vi "SaveImagesFromArray (SubVI).vi"(8 "error in (no error)":errorcluster, 9 "Array of Images":T1[](array[typedef]), 10 "XY Camera Coordinates":dbl[][](array[numeric]), 11 "Path to save collected images":path=path "E:/XYZstage+Camera_CollectedImages/12-17-2016/images") -> (0 "error out":errorcluster)   [LabVIEW 2016]
uses:
  <vilib>/vision/Image Controls.llb/IMAQ Image.ctl
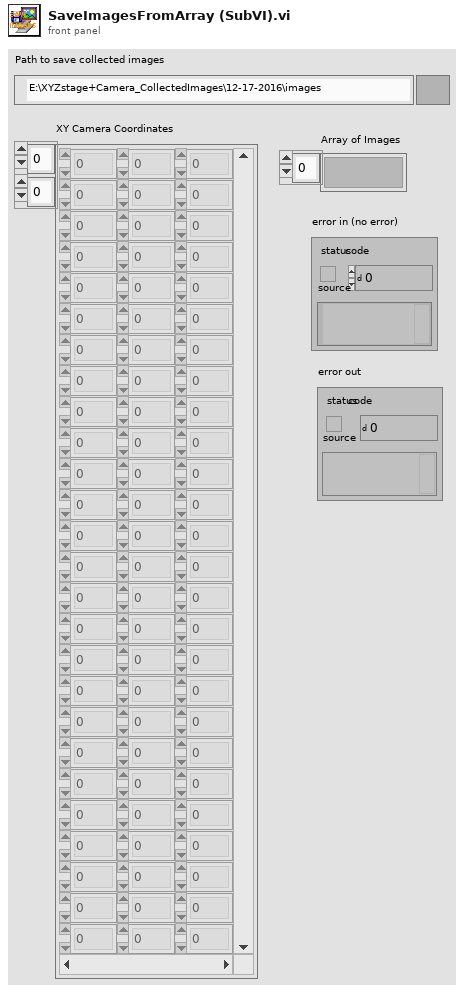
[diagram p1: front panel]
types:
  T1 = typedef "IMAQ Image.ctl" = refnum<image>
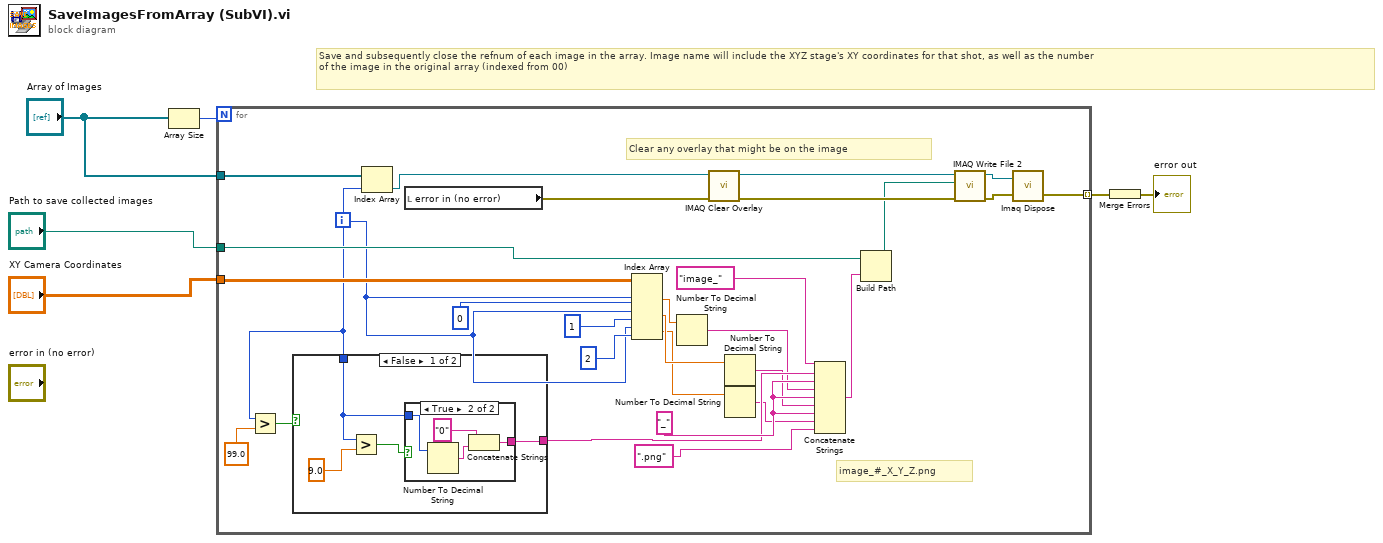
[diagram p0: block diagram]
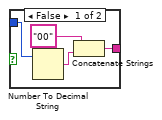
[diagram p2: hidden frame]
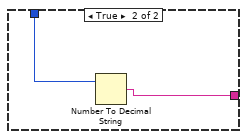
[diagram p3: hidden frame]
diagram:
  # "Save and subsequently close the refnum of each image in the array. Image name will include the XYZ stage's XY coordinates for that shot, as well as the number\nof the image in the original array (indexed from 00)"
  n1 = Array Size(array="Array of Images") -> (size(s)=w3:i32)
  n2 = for {
    N: w3 -> [_]
    tunnel: "Array of Images" -> [w34]
    tunnel: "Path to save collected images" -> [w27]
    tunnel: "XY Camera Coordinates" -> [w26]
    tunnel: [w23] -> w2 mode=indexing
    i -> [w7]
    w14 = "_" ("string")
    # "image_#_X_Y_Z.png"
    # "Clear any overlay that might be on the image"
    n3 = Greater?(x=w7, y=99.0) -> (0:w9:bool)
    n4 = case shown="False" w9 {
      tunnel: w7 -> [w35 w48]
      tunnel: [w37 w47] -> w13
      frame False {
        n5 = Greater?(x=w35, y=9.0) -> (0:w36:bool)
        n6 = case shown="True" w36 {
          tunnel: [w40 w43] -> w37
          tunnel: w35 -> [w39 w44]
          frame False {
            n7 = Number To Decimal String(number=w39) -> (decimal integer string=w42:string)  [unwired: 1 in]
            n8 = Concatenate Strings("00" ("string"), w42) -> (w40:string)
          }
          frame True {
            n9 = Number To Decimal String(number=w44) -> (decimal integer string=w46:string)  [unwired: 1 in]
            n10 = Concatenate Strings("0" ("string"), w46) -> (w43:string)
          }
        }
      }
      frame True {
        n11 = Number To Decimal String(number=w48) -> (decimal integer string=w47:string)  [unwired: 1 in]
      }
    }
    n12 = Index Array(array=w34, index=w7) -> (element=w22:T1)
    n13 = local read "error in (no error)"() -> (w21:errorcluster)
    n14 = Index Array(array=w26, index (row) #1=w7, index (col) #1=0 ("disabled index (col)"), index (row) #2=w7, index (col) #2=1 ("disabled index (col)"), index (row) #3=w7, index (col) #3=2 ("index (col)")) -> (element #1=w30:dbl, element #2=w28:dbl, element #3=w15:dbl)
    n15 = Number To Decimal String(number=w30) -> (decimal integer string=w12:string)  [unwired: 1 in]
    n16 = call "IMAQ Clear Overlay"("error in (no error)"=w21, "Image"=w22) -> ("error out"=w20:errorcluster, "Image Out"=w19:T1)  [unwired: 8 in]
    n17 = Number To Decimal String(number=w28) -> (decimal integer string=w11:string)  [unwired: 1 in]
    n18 = Number To Decimal String(number=w15) -> (decimal integer string=w10:string)  [unwired: 1 in]
    n19 = Concatenate Strings("image_" ("string"), w13, w14, w12, w14, w11, w14, w10, ".png" ("string")) -> (w33:string)
    n20 = Build Path(base path=w27, name or relative path=w33) -> (appended path=w18:path)
    n21 = call-poly "IMAQ Write File 2"("error in (no error)"=w20, "File Path"=w18, "Image"=w19) -> ("error out"=w24:errorcluster, "Image Out (duplicate)"=w25:T1)  [unwired: 7 in]
    n22 = call "Imaq Dispose"("Image"=w25, "error in (no error)"=w24) -> ("error out"=w23:errorcluster)  [unwired: 4 in]
  }
  n23 = Merge Errors(w2) -> (→"error out":errorcluster)
